vi "Sort File List.vi"(8 "error in":errorcluster, 11 "Peer Review":refnum<class "Peer Review.lvclass">) -> (0 "error out":errorcluster, 2 "Sorted File List":T1[](array[typedef]))   [LabVIEW 2020, in "Peer Review.lvclass"]
uses:
  Peer Review.lvclass
  TypeDefs/File Info.ctl
  TypeDefs/File State.ctl
  TypeDefs/VI Type.ctl
  Peer Review.lvclass/Peer Review.ctl
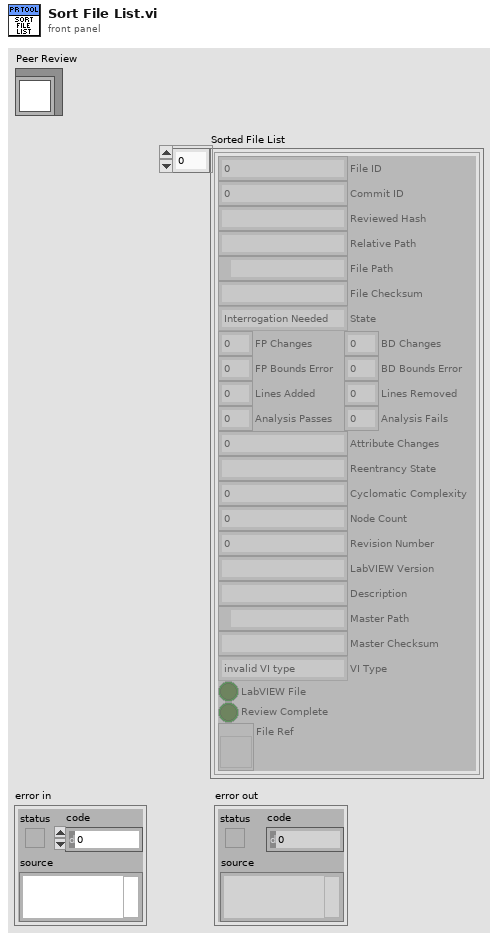
[diagram p1: front panel]
types:
  T1 = typedef "Peer Review.lvclass/File Info.ctl" = cluster{"File ID":i32, "Commit ID":i32, "Reviewed Hash":string, "Relative Path":string, "File Path":path, "File Checksum":string, "State":T2, "FP Changes":i32, "BD Changes":i32, "FP Bounds Error":dbl, "BD Bounds Error":dbl, "Lines Added":i32, "Lines Removed":i32, "Analysis Passes":i32, "Analysis Fails":i32, "Attribute Changes":i32, "Reentrancy State":string, "Cyclomatic Complexity":i32, "Node Count":i32, "Revision Number":u32, "LabVIEW Version":string, "Description":string, "Master Path":path, "Master Checksum":string, "VI Type":T3, "LabVIEW File":bool, "Review Complete":bool, "File Ref":refnum<vi>}
  T2 = typedef "Peer Review.lvclass/File State.ctl" = enum16{"Interrogation Needed", "Modified", "Deleted", "Added", "Matches Previous", "No Changes", "Moved"}
  T3 = typedef "Peer Review.lvclass/VI Type.ctl" = enum32{"invalid VI type", "Standard VI", "Control VI", "Global VI", "Polymorphic VI", "Configuration VI", "SubSystem", "Facade VI", "Method VI", "Statechart Diagram VI"}
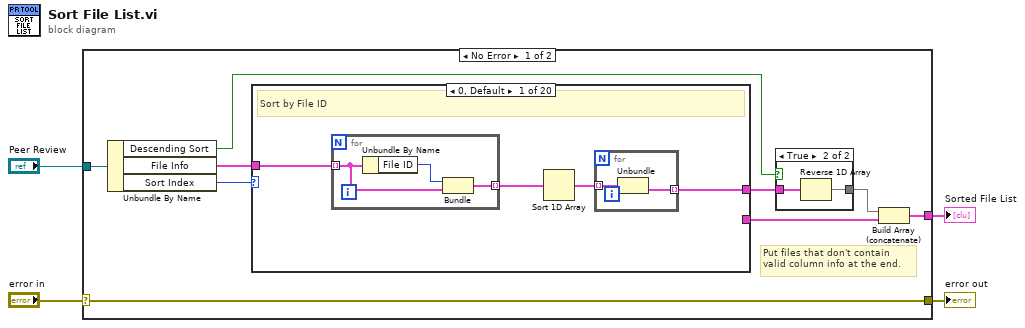
[diagram p0: block diagram]
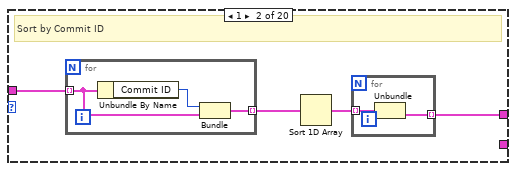
[diagram p3: hidden frame]
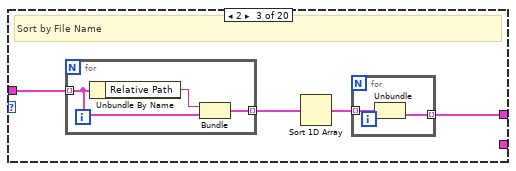
[diagram p4: hidden frame]
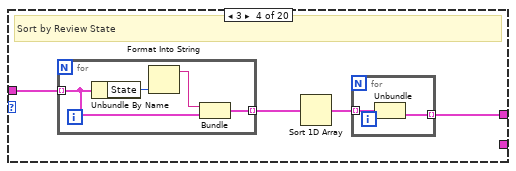
[diagram p5: hidden frame]
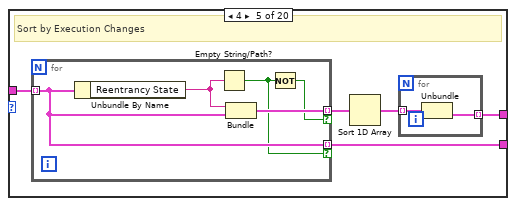
[diagram p6: hidden frame]
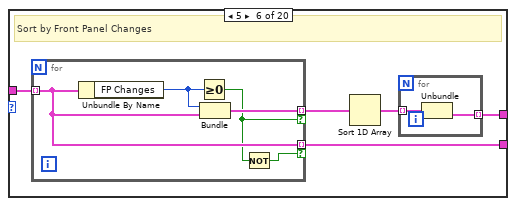
[diagram p7: hidden frame]
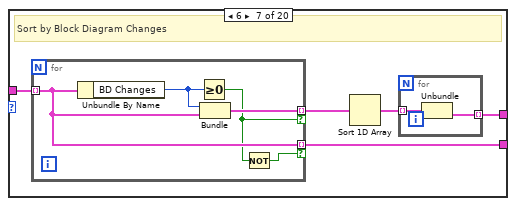
[diagram p8: hidden frame]
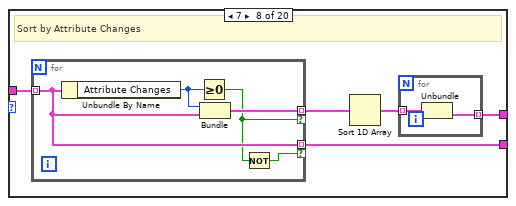
[diagram p9: hidden frame]
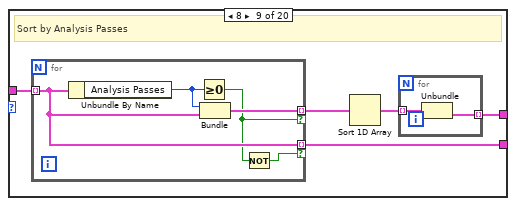
[diagram p10: hidden frame]
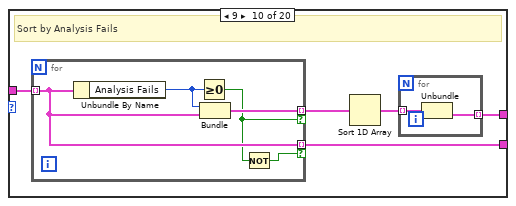
[diagram p11: hidden frame]
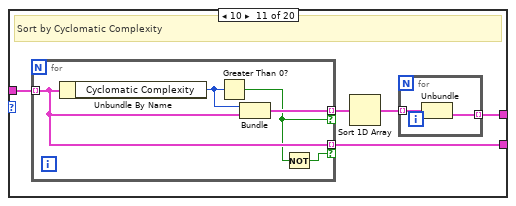
[diagram p12: hidden frame]
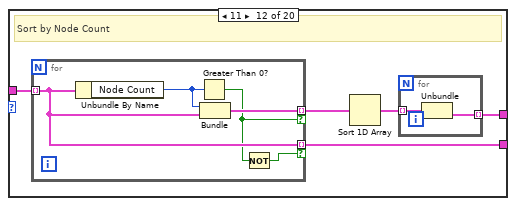
[diagram p13: hidden frame]
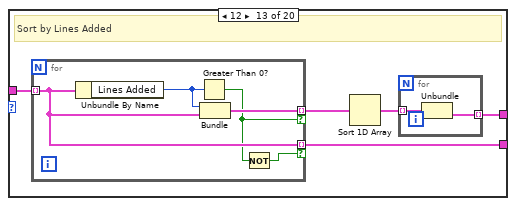
[diagram p14: hidden frame]
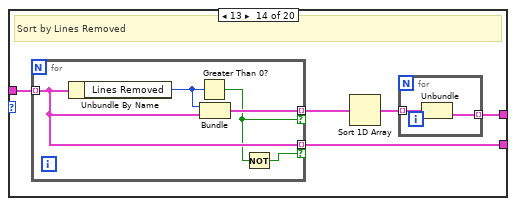
[diagram p15: hidden frame]
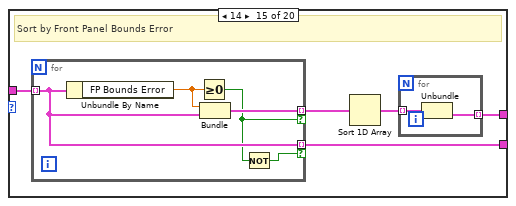
[diagram p16: hidden frame]
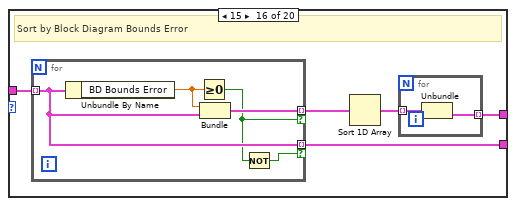
[diagram p17: hidden frame]
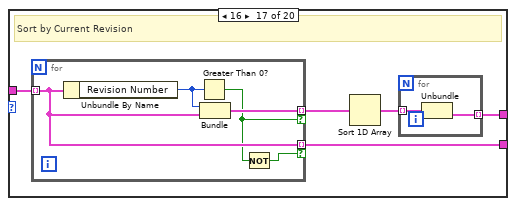
[diagram p18: hidden frame]
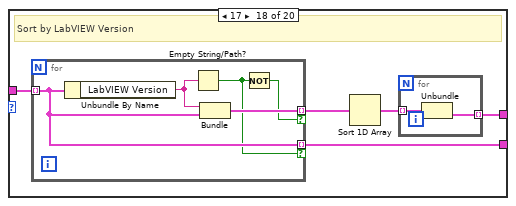
[diagram p19: hidden frame]
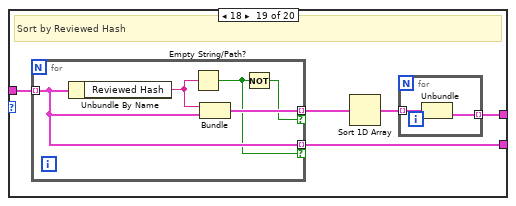
[diagram p20: hidden frame]
diagram:
  n1 = case shown="No Error" "error in" {
    selector: "error in" -> [w10 w246]
    tunnel: [w5 _] -> w4
    tunnel: "Peer Review" -> [w13 _]
    tunnel: [w10 w246] -> w2
    frame No Error {
      # "Put files that don't contain\nvalid column info at the end."
      n2 = Unbundle By Name(w13) -> ("Descending Sort"=w8:bool, "File Info"=w12:T1[], "Sort Index"=w11:i32)
      n3 = case shown="0, Default" w11 {
        tunnel: w12 -> [w20 w29 w38 w47 w58 w70 w82 w94 w106 w118 w130 w142 w154 w166 w178 w190 w202 w214 w226 w238]
        tunnel: [w17 w26 w35 w44 w55 w67 w79 w91 w103 w115 w127 w139 w151 w163 w175 w187 w199 w211 w223 w235] -> w9
        tunnel: [_ _ _ _ w54 w66 w78 w90 w102 w114 w126 w138 w150 w162 w174 w186 w198 w210 w222 w234] -> w7
        frame 0, Default {
          # "Sort by File ID"
          n4 = for {
            tunnel: w20 -> [w24] mode=indexing
            tunnel: [w23] -> w19 mode=indexing
            n5 = Unbundle By Name(w24) -> ("File ID"=w25:i32)
            n6 = Bundle("File ID"=w25, w24) -> (w23:cluster{"File ID":i32, T1})  [unwired: 1 in]
          }
          n7 = Sort 1D Array(array=w19) -> (sorted array=w18:cluster{"File ID":i32, T1}[])
          n8 = for {
            tunnel: w18 -> [w22] mode=indexing
            tunnel: [w21] -> w17 mode=indexing
            n9 = Unbundle(w22) -> (w21:T1)  [unwired: 1 out]
          }
        }
        frame 1 {
          # "Sort by Commit ID"
          n10 = for {
            tunnel: w29 -> [w33] mode=indexing
            tunnel: [w32] -> w28 mode=indexing
            n11 = Unbundle By Name(w33) -> ("Commit ID"=w34:i32)
            n12 = Bundle("Commit ID"=w34, w33) -> (w32:cluster{"Commit ID":i32, T1})  [unwired: 1 in]
          }
          n13 = Sort 1D Array(array=w28) -> (sorted array=w27:cluster{"Commit ID":i32, T1}[])
          n14 = for {
            tunnel: w27 -> [w31] mode=indexing
            tunnel: [w30] -> w26 mode=indexing
            n15 = Unbundle(w31) -> (w30:T1)  [unwired: 1 out]
          }
        }
        frame 2 {
          # "Sort by File Name"
          n16 = for {
            tunnel: w38 -> [w42] mode=indexing
            tunnel: [w41] -> w37 mode=indexing
            n17 = Unbundle By Name(w42) -> ("Relative Path"=w43:string)
            n18 = Bundle("Relative Path"=w43, w42) -> (w41:cluster{"Relative Path":string, T1})  [unwired: 1 in]
          }
          n19 = Sort 1D Array(array=w37) -> (sorted array=w36:cluster{"Relative Path":string, T1}[])
          n20 = for {
            tunnel: w36 -> [w40] mode=indexing
            tunnel: [w39] -> w35 mode=indexing
            n21 = Unbundle(w40) -> (w39:T1)  [unwired: 1 out]
          }
        }
        frame 3 {
          # "Sort by Review State"
          n22 = for {
            tunnel: w47 -> [w53] mode=indexing
            tunnel: [w52] -> w46 mode=indexing
            n23 = Unbundle By Name(w53) -> ("State"=w51:T2)
            n24 = Format Into String(w51) -> (resulting string=w50:string)  [unwired: 3 in, 1 out]
            n25 = Bundle(w50, w53) -> (w52:cluster{string, T1})  [unwired: 1 in]
          }
          n26 = Sort 1D Array(array=w46) -> (sorted array=w45:cluster{string, T1}[])
          n27 = for {
            tunnel: w45 -> [w49] mode=indexing
            tunnel: [w48] -> w44 mode=indexing
            n28 = Unbundle(w49) -> (w48:T1)  [unwired: 1 out]
          }
        }
        frame 4 {
          # "Sort by Execution Changes"
          n29 = for {
            tunnel: w58 -> [w64] mode=indexing
            tunnel: [w65] -> w57 mode=indexing if=w62
            tunnel: [w64] -> w54 mode=indexing if=w61
            n30 = Unbundle By Name(w64) -> ("Reentrancy State"=w63:string)
            n31 = Empty String/Path?(string/path=w63) -> (empty?=w61:bool)
            n32 = Bundle("Reentrancy State"=w63, w64) -> (w65:cluster{"Reentrancy State":string, T1})  [unwired: 1 in]
            n33 = Not(x=w61) -> (.not. x?=w62:bool)
          }
          n34 = Sort 1D Array(array=w57) -> (sorted array=w56:cluster{"Reentrancy State":string, T1}[])
          n35 = for {
            tunnel: w56 -> [w60] mode=indexing
            tunnel: [w59] -> w55 mode=indexing
            n36 = Unbundle(w60) -> (w59:T1)  [unwired: 1 out]
          }
        }
        frame 5 {
          # "Sort by Front Panel Changes"
          n37 = for {
            tunnel: w70 -> [w75] mode=indexing
            tunnel: [w77] -> w69 mode=indexing if=w74
            tunnel: [w75] -> w66 mode=indexing if=w73
            n38 = Unbundle By Name(w75) -> ("FP Changes"=w76:i32)
            n39 = Greater Or Equal To 0?(x=w76) -> (x >= 0?=w74:bool)
            n40 = Bundle("FP Changes"=w76, w75) -> (w77:cluster{"FP Changes":i32, T1})  [unwired: 1 in]
            n41 = Not(x=w74) -> (.not. x?=w73:bool)
          }
          n42 = Sort 1D Array(array=w69) -> (sorted array=w68:cluster{"FP Changes":i32, T1}[])
          n43 = for {
            tunnel: w68 -> [w72] mode=indexing
            tunnel: [w71] -> w67 mode=indexing
            n44 = Unbundle(w72) -> (w71:T1)  [unwired: 1 out]
          }
        }
        frame 6 {
          # "Sort by Block Diagram Changes"
          n45 = for {
            tunnel: w82 -> [w87] mode=indexing
            tunnel: [w89] -> w81 mode=indexing if=w86
            tunnel: [w87] -> w78 mode=indexing if=w85
            n46 = Unbundle By Name(w87) -> ("BD Changes"=w88:i32)
            n47 = Greater Or Equal To 0?(x=w88) -> (x >= 0?=w86:bool)
            n48 = Bundle("BD Changes"=w88, w87) -> (w89:cluster{"BD Changes":i32, T1})  [unwired: 1 in]
            n49 = Not(x=w86) -> (.not. x?=w85:bool)
          }
          n50 = Sort 1D Array(array=w81) -> (sorted array=w80:cluster{"BD Changes":i32, T1}[])
          n51 = for {
            tunnel: w80 -> [w84] mode=indexing
            tunnel: [w83] -> w79 mode=indexing
            n52 = Unbundle(w84) -> (w83:T1)  [unwired: 1 out]
          }
        }
        frame 7 {
          # "Sort by Attribute Changes"
          n53 = for {
            tunnel: w94 -> [w99] mode=indexing
            tunnel: [w101] -> w93 mode=indexing if=w98
            tunnel: [w99] -> w90 mode=indexing if=w97
            n54 = Unbundle By Name(w99) -> ("Attribute Changes"=w100:i32)
            n55 = Greater Or Equal To 0?(x=w100) -> (x >= 0?=w98:bool)
            n56 = Bundle("Attribute Changes"=w100, w99) -> (w101:cluster{"Attribute Changes":i32, T1})  [unwired: 1 in]
            n57 = Not(x=w98) -> (.not. x?=w97:bool)
          }
          n58 = Sort 1D Array(array=w93) -> (sorted array=w92:cluster{"Attribute Changes":i32, T1}[])
          n59 = for {
            tunnel: w92 -> [w96] mode=indexing
            tunnel: [w95] -> w91 mode=indexing
            n60 = Unbundle(w96) -> (w95:T1)  [unwired: 1 out]
          }
        }
        frame 8 {
          # "Sort by Analysis Passes"
          n61 = for {
            tunnel: w106 -> [w111] mode=indexing
            tunnel: [w113] -> w105 mode=indexing if=w110
            tunnel: [w111] -> w102 mode=indexing if=w109
            n62 = Unbundle By Name(w111) -> ("Analysis Passes"=w112:i32)
            n63 = Greater Or Equal To 0?(x=w112) -> (x >= 0?=w110:bool)
            n64 = Bundle("Analysis Passes"=w112, w111) -> (w113:cluster{"Analysis Passes":i32, T1})  [unwired: 1 in]
            n65 = Not(x=w110) -> (.not. x?=w109:bool)
          }
          n66 = Sort 1D Array(array=w105) -> (sorted array=w104:cluster{"Analysis Passes":i32, T1}[])
          n67 = for {
            tunnel: w104 -> [w108] mode=indexing
            tunnel: [w107] -> w103 mode=indexing
            n68 = Unbundle(w108) -> (w107:T1)  [unwired: 1 out]
          }
        }
        frame 9 {
          # "Sort by Analysis Fails"
          n69 = for {
            tunnel: w118 -> [w123] mode=indexing
            tunnel: [w125] -> w117 mode=indexing if=w122
            tunnel: [w123] -> w114 mode=indexing if=w121
            n70 = Unbundle By Name(w123) -> ("Analysis Fails"=w124:i32)
            n71 = Greater Or Equal To 0?(x=w124) -> (x >= 0?=w122:bool)
            n72 = Bundle("Analysis Fails"=w124, w123) -> (w125:cluster{"Analysis Fails":i32, T1})  [unwired: 1 in]
            n73 = Not(x=w122) -> (.not. x?=w121:bool)
          }
          n74 = Sort 1D Array(array=w117) -> (sorted array=w116:cluster{"Analysis Fails":i32, T1}[])
          n75 = for {
            tunnel: w116 -> [w120] mode=indexing
            tunnel: [w119] -> w115 mode=indexing
            n76 = Unbundle(w120) -> (w119:T1)  [unwired: 1 out]
          }
        }
        frame 10 {
          # "Sort by Cyclomatic Complexity"
          n77 = for {
            tunnel: w130 -> [w135] mode=indexing
            tunnel: [w137] -> w129 mode=indexing if=w134
            tunnel: [w135] -> w126 mode=indexing if=w133
            n78 = Unbundle By Name(w135) -> ("Cyclomatic Complexity"=w136:i32)
            n79 = Greater Than 0?(x=w136) -> (x > 0?=w134:bool)
            n80 = Bundle("Cyclomatic Complexity"=w136, w135) -> (w137:cluster{"Cyclomatic Complexity":i32, T1})  [unwired: 1 in]
            n81 = Not(x=w134) -> (.not. x?=w133:bool)
          }
          n82 = Sort 1D Array(array=w129) -> (sorted array=w128:cluster{"Cyclomatic Complexity":i32, T1}[])
          n83 = for {
            tunnel: w128 -> [w132] mode=indexing
            tunnel: [w131] -> w127 mode=indexing
            n84 = Unbundle(w132) -> (w131:T1)  [unwired: 1 out]
          }
        }
        frame 11 {
          # "Sort by Node Count"
          n85 = for {
            tunnel: w142 -> [w147] mode=indexing
            tunnel: [w149] -> w141 mode=indexing if=w146
            tunnel: [w147] -> w138 mode=indexing if=w145
            n86 = Unbundle By Name(w147) -> ("Node Count"=w148:i32)
            n87 = Greater Than 0?(x=w148) -> (x > 0?=w146:bool)
            n88 = Bundle("Node Count"=w148, w147) -> (w149:cluster{"Node Count":i32, T1})  [unwired: 1 in]
            n89 = Not(x=w146) -> (.not. x?=w145:bool)
          }
          n90 = Sort 1D Array(array=w141) -> (sorted array=w140:cluster{"Node Count":i32, T1}[])
          n91 = for {
            tunnel: w140 -> [w144] mode=indexing
            tunnel: [w143] -> w139 mode=indexing
            n92 = Unbundle(w144) -> (w143:T1)  [unwired: 1 out]
          }
        }
        frame 12 {
          # "Sort by Lines Added"
          n93 = for {
            tunnel: w154 -> [w159] mode=indexing
            tunnel: [w161] -> w153 mode=indexing if=w158
            tunnel: [w159] -> w150 mode=indexing if=w157
            n94 = Unbundle By Name(w159) -> ("Lines Added"=w160:i32)
            n95 = Greater Than 0?(x=w160) -> (x > 0?=w158:bool)
            n96 = Bundle("Lines Added"=w160, w159) -> (w161:cluster{"Lines Added":i32, T1})  [unwired: 1 in]
            n97 = Not(x=w158) -> (.not. x?=w157:bool)
          }
          n98 = Sort 1D Array(array=w153) -> (sorted array=w152:cluster{"Lines Added":i32, T1}[])
          n99 = for {
            tunnel: w152 -> [w156] mode=indexing
            tunnel: [w155] -> w151 mode=indexing
            n100 = Unbundle(w156) -> (w155:T1)  [unwired: 1 out]
          }
        }
        frame 13 {
          # "Sort by Lines Removed"
          n101 = for {
            tunnel: w166 -> [w171] mode=indexing
            tunnel: [w173] -> w165 mode=indexing if=w170
            tunnel: [w171] -> w162 mode=indexing if=w169
            n102 = Unbundle By Name(w171) -> ("Lines Removed"=w172:i32)
            n103 = Greater Than 0?(x=w172) -> (x > 0?=w170:bool)
            n104 = Bundle("Lines Removed"=w172, w171) -> (w173:cluster{"Lines Removed":i32, T1})  [unwired: 1 in]
            n105 = Not(x=w170) -> (.not. x?=w169:bool)
          }
          n106 = Sort 1D Array(array=w165) -> (sorted array=w164:cluster{"Lines Removed":i32, T1}[])
          n107 = for {
            tunnel: w164 -> [w168] mode=indexing
            tunnel: [w167] -> w163 mode=indexing
            n108 = Unbundle(w168) -> (w167:T1)  [unwired: 1 out]
          }
        }
        frame 14 {
          # "Sort by Front Panel Bounds Error"
          n109 = for {
            tunnel: w178 -> [w183] mode=indexing
            tunnel: [w185] -> w177 mode=indexing if=w182
            tunnel: [w183] -> w174 mode=indexing if=w181
            n110 = Unbundle By Name(w183) -> ("FP Bounds Error"=w184:dbl)
            n111 = Greater Or Equal To 0?(x=w184) -> (x >= 0?=w182:bool)
            n112 = Bundle("FP Bounds Error"=w184, w183) -> (w185:cluster{"FP Bounds Error":dbl, T1})  [unwired: 1 in]
            n113 = Not(x=w182) -> (.not. x?=w181:bool)
          }
          n114 = Sort 1D Array(array=w177) -> (sorted array=w176:cluster{"FP Bounds Error":dbl, T1}[])
          n115 = for {
            tunnel: w176 -> [w180] mode=indexing
            tunnel: [w179] -> w175 mode=indexing
            n116 = Unbundle(w180) -> (w179:T1)  [unwired: 1 out]
          }
        }
        frame 15 {
          # "Sort by Block Diagram Bounds Error"
          n117 = for {
            tunnel: w190 -> [w195] mode=indexing
            tunnel: [w197] -> w189 mode=indexing if=w194
            tunnel: [w195] -> w186 mode=indexing if=w193
            n118 = Unbundle By Name(w195) -> ("BD Bounds Error"=w196:dbl)
            n119 = Greater Or Equal To 0?(x=w196) -> (x >= 0?=w194:bool)
            n120 = Bundle("BD Bounds Error"=w196, w195) -> (w197:cluster{"BD Bounds Error":dbl, T1})  [unwired: 1 in]
            n121 = Not(x=w194) -> (.not. x?=w193:bool)
          }
          n122 = Sort 1D Array(array=w189) -> (sorted array=w188:cluster{"BD Bounds Error":dbl, T1}[])
          n123 = for {
            tunnel: w188 -> [w192] mode=indexing
            tunnel: [w191] -> w187 mode=indexing
            n124 = Unbundle(w192) -> (w191:T1)  [unwired: 1 out]
          }
        }
        frame 16 {
          # "Sort by Current Revision"
          n125 = for {
            tunnel: w202 -> [w207] mode=indexing
            tunnel: [w209] -> w201 mode=indexing if=w206
            tunnel: [w207] -> w198 mode=indexing if=w205
            n126 = Unbundle By Name(w207) -> ("Revision Number"=w208:u32)
            n127 = Greater Than 0?(x=w208) -> (x > 0?=w206:bool)
            n128 = Bundle("Revision Number"=w208, w207) -> (w209:cluster{"Revision Number":u32, T1})  [unwired: 1 in]
            n129 = Not(x=w206) -> (.not. x?=w205:bool)
          }
          n130 = Sort 1D Array(array=w201) -> (sorted array=w200:cluster{"Revision Number":u32, T1}[])
          n131 = for {
            tunnel: w200 -> [w204] mode=indexing
            tunnel: [w203] -> w199 mode=indexing
            n132 = Unbundle(w204) -> (w203:T1)  [unwired: 1 out]
          }
        }
        frame 17 {
          # "Sort by LabVIEW Version"
          n133 = for {
            tunnel: w214 -> [w220] mode=indexing
            tunnel: [w221] -> w213 mode=indexing if=w218
            tunnel: [w220] -> w210 mode=indexing if=w217
            n134 = Unbundle By Name(w220) -> ("LabVIEW Version"=w219:string)
            n135 = Empty String/Path?(string/path=w219) -> (empty?=w217:bool)
            n136 = Bundle("LabVIEW Version"=w219, w220) -> (w221:cluster{"LabVIEW Version":string, T1})  [unwired: 1 in]
            n137 = Not(x=w217) -> (.not. x?=w218:bool)
          }
          n138 = Sort 1D Array(array=w213) -> (sorted array=w212:cluster{"LabVIEW Version":string, T1}[])
          n139 = for {
            tunnel: w212 -> [w216] mode=indexing
            tunnel: [w215] -> w211 mode=indexing
            n140 = Unbundle(w216) -> (w215:T1)  [unwired: 1 out]
          }
        }
        frame 18 {
          # "Sort by Reviewed Hash"
          n141 = for {
            tunnel: w226 -> [w232] mode=indexing
            tunnel: [w233] -> w225 mode=indexing if=w230
            tunnel: [w232] -> w222 mode=indexing if=w229
            n142 = Unbundle By Name(w232) -> ("Reviewed Hash"=w231:string)
            n143 = Empty String/Path?(string/path=w231) -> (empty?=w229:bool)
            n144 = Bundle("Reviewed Hash"=w231, w232) -> (w233:cluster{"Reviewed Hash":string, T1})  [unwired: 1 in]
            n145 = Not(x=w229) -> (.not. x?=w230:bool)
          }
          n146 = Sort 1D Array(array=w225) -> (sorted array=w224:cluster{"Reviewed Hash":string, T1}[])
          n147 = for {
            tunnel: w224 -> [w228] mode=indexing
            tunnel: [w227] -> w223 mode=indexing
            n148 = Unbundle(w228) -> (w227:T1)  [unwired: 1 out]
          }
        }
        frame 19 {
          # "Sort by Master Path"
          n149 = for {
            tunnel: w238 -> [w244] mode=indexing
            tunnel: [w245] -> w237 mode=indexing if=w241
            tunnel: [w244] -> w234 mode=indexing if=w243
            n150 = Unbundle By Name(w244) -> ("Master Path"=w242:path)
            n151 = call <vilib>:"Is Path and Not Empty.vi"("path"=w242) -> ("Is Path and Not Empty?"=w241:bool)  [unwired: 4 in]
            n152 = Bundle("Master Path"=w242, w244) -> (w245:cluster{"Master Path":path, T1})  [unwired: 1 in]
            n153 = Not(x=w241) -> (.not. x?=w243:bool)
          }
          n154 = Sort 1D Array(array=w237) -> (sorted array=w236:cluster{"Master Path":path, T1}[])
          n155 = for {
            tunnel: w236 -> [w240] mode=indexing
            tunnel: [w239] -> w235 mode=indexing
            n156 = Unbundle(w240) -> (w239:T1)  [unwired: 1 out]
          }
        }
      }
      n157 = case shown="True" w8 {
        tunnel: w9 -> [w14 w16]
        tunnel: [w14 w15] -> w6
        frame False {
        }
        frame True {
          n158 = Reverse 1D Array(array=w16) -> (reversed array=w15:T1[])
        }
      }
      n159 = Build Array (concatenate)(w6, w7) -> (w5:T1[])
    }
    frame Error {
    }
  }
  "error out" <- w2
  "Sorted File List" <- w4
